vi "class_data.vi"() -> ()   [LabVIEW 2010, in "FPGAWrapperAK101022Resonance.lvclass"]
uses:
  FPGAWrapperAK101022Resonance.lvclass
  scan_specification_cluster.ctl
  grabber/config_data_cluster.ctl
panel:
  out "configuration writer endpoint":refnum<k21>
  in  "# of callers":i32
  in  "scan specification refnum":refnum<k21>
  in  "FPGA buffer overflow refnum":refnum<k21>
  out "terminating?":bool
  in  "data  reader endpoint":refnum<k21>
  in  "command writer endpoint":refnum<k21>
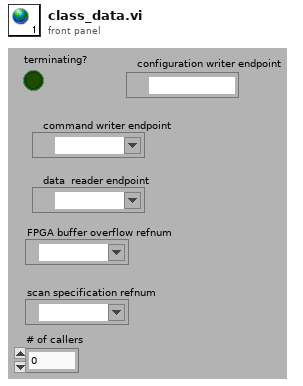
[diagram p1: front panel]
diagram:
